vi "Events Trigger.vi"() -> ()   [LabVIEW 2014]
panel:
  in  "Click (Event)":bool
  in  "Click (no Event)":bool
  out "teste":dbl
  in  "Numeric":dbl
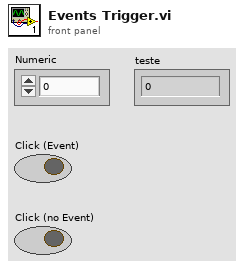
[diagram p1: front panel]
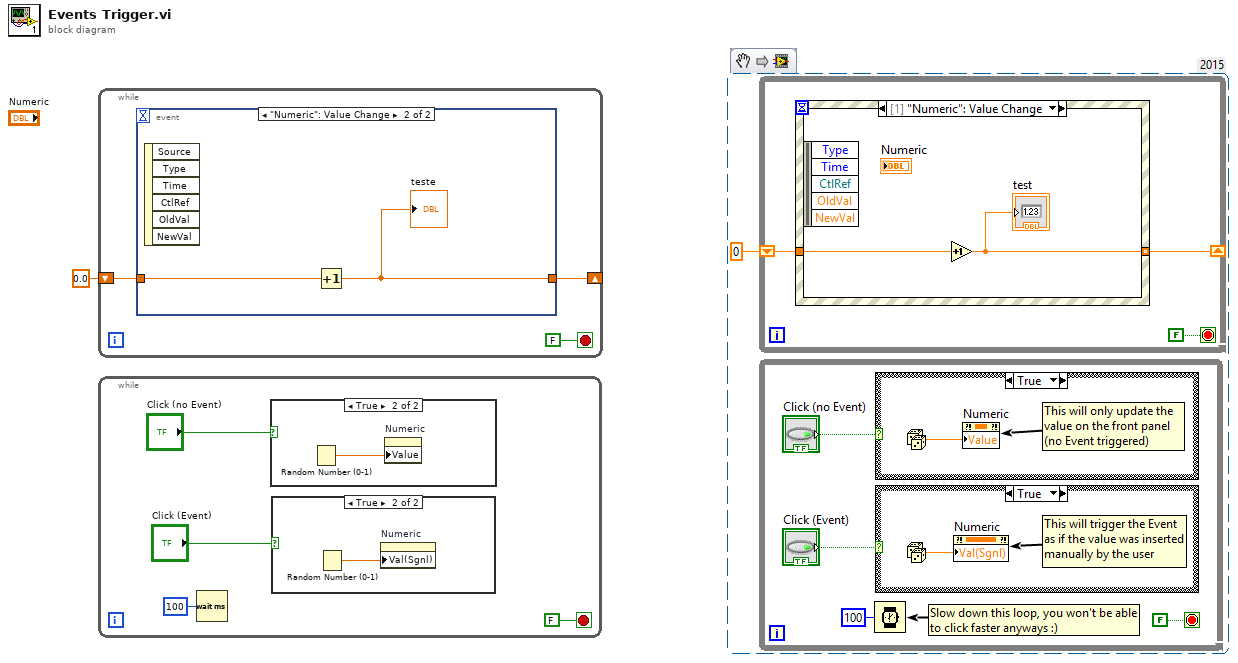
[diagram p0: block diagram]
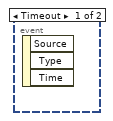
[diagram p4: hidden frame]
diagram:
  n1 = while {
    shift-right: [w3] -> _
    shift-left: 0.0 -> [w4]
    stop <- FALSE stop-if-true
    n2 = event shown="[1] \"Numeric\": Value Change" {
      selector: _ -> [_ _]
      dyn-events: _ -> [_ _]
      timeout: _ -> [_ _]
      tunnel: w4 -> [_ w6]
      tunnel: [_ w5] -> w3
      event Timeout {
        n3 = event-data() -> ()  [unwired: 1 in, 3 out]
      }
      event "Numeric": Value Change {
        n4 = event-data() -> ()  [unwired: 1 in, 6 out]
        n5 = Increment(x=w6) -> (x+1=w5:dbl)
        "teste" <- w5
      }
    }
  }
  n6 = while {
    stop <- FALSE stop-if-true
    n7 = Wait (ms)(milliseconds to wait=u32 100) -> ()  [unwired: 1 out]
    n8 = case shown="True" "Click (no Event)" {
      frame False {
      }
      frame True {
        n9 = Random Number (0-1)() -> (number: 0 to 1=w12:dbl)
        n10 = property on="Numeric" class="DigNum (strict)"("Value"=w12) -> ()  [unwired: 2 in, 2 out]
      }
    }
    n11 = case shown="True" "Click (Event)" {
      frame False {
      }
      frame True {
        n12 = Random Number (0-1)() -> (number: 0 to 1=w11:dbl)
        n13 = property on="Numeric" class="DigNum (strict)"("Val(Sgnl)"=w11) -> ()  [unwired: 2 in, 2 out]
      }
    }
  }
